vi "monostepgf.vi"(0 "Wait Between Steps(ms)":u32=8, 1 "Steps":i32=1, 2 "Direction":string, 3 "address":i16 format="%.0x") -> ()   [LabVIEW 2010]
uses:
  <vilib>/Platform/portaccess.llb/Out Port32.vi
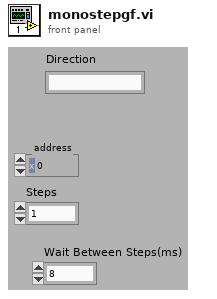
[diagram p1: front panel]
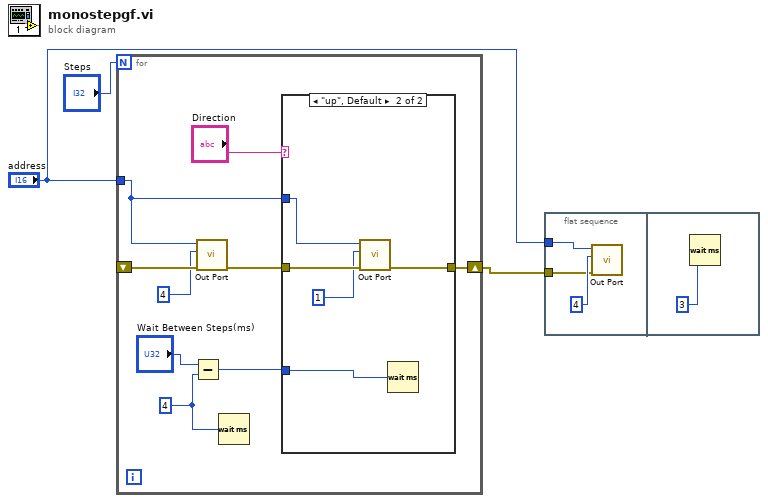
[diagram p0: block diagram]
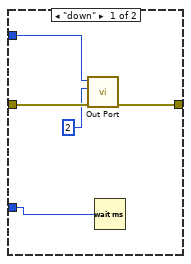
[diagram p2: hidden frame]
diagram:
  n1 = for {
    N: "Steps" -> [_]
    tunnel: "address" -> [w11]
    shift-right: [w9] -> w1
    shift-left: _ -> [w8]
    w4 = u32 4
    n2 = Subtract(x="Wait Between Steps(ms)", y=w4) -> (x-y=w5:u32)
    n3 = call-poly <vilib>:"Out Port.vi"("error in (no error)"=w8, "write value"=4, "address"=w11) -> ("error out"=w10:errorcluster)  [unwired: 6 in]
    n4 = Wait (ms)(milliseconds to wait=w4) -> ()  [unwired: 1 out]
    n5 = case shown="\"up\", Default" "Direction" {
      tunnel: w11 -> [w17 w22]
      tunnel: w10 -> [w16 w21]
      tunnel: [w15 w20] -> w9
      tunnel: w5 -> [w13 w18]
      frame "down" {
        n6 = call-poly <vilib>:"Out Port.vi"("error in (no error)"=w16, "write value"=2, "address"=w17) -> ("error out"=w15:errorcluster)  [unwired: 6 in]
        n7 = Wait (ms)(milliseconds to wait=w13) -> ()  [unwired: 1 out]
      }
      frame "up", Default {
        n8 = call-poly <vilib>:"Out Port.vi"("error in (no error)"=w21, "write value"=1, "address"=w22) -> ("error out"=w20:errorcluster)  [unwired: 6 in]
        n9 = Wait (ms)(milliseconds to wait=w18) -> ()  [unwired: 1 out]
      }
    }
  }
  n10 = flat-sequence {
    tunnel: "address" -> [w24]
    tunnel: w1 -> [w23]
    frame #0 {
      n11 = call-poly <vilib>:"Out Port.vi"("error in (no error)"=w23, "write value"=4, "address"=w24) -> ()  [unwired: 6 in, 1 out]
    }
    frame #1 {
      n12 = Wait (ms)(milliseconds to wait=u32 3) -> ()  [unwired: 1 out]
    }
  }
